vi "Init Platform Plugins.vi"(8 "error in (no error)":errorcluster, 11 "picoG in":refnum<class "picoG.lvclass">) -> (0 "error out":errorcluster, 3 "picoG out":refnum<class "picoG.lvclass">)   [LabVIEW 2020, in "PicoG-App.lvlib" / "picoG.lvclass"]
uses:
  picoG.lvclass
  picoG.lvclass/picoG.ctl
  Builds/picoG/ppl/PicoG-Core.lvlibp/PicoG-Processor/PicoG-Core/PlatformPluginManager/PlatformPluginManager.lvclass
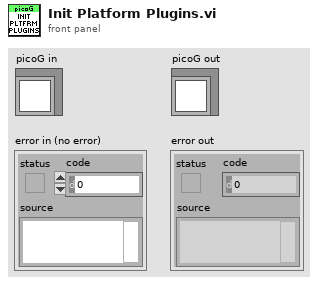
[diagram p1: front panel]
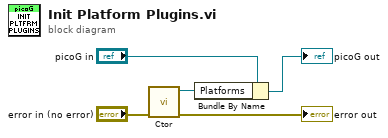
[diagram p0: block diagram]
diagram:
  n1 = call "Ctor.vi"("error in (no error)"="error in (no error)") -> ("error out"=→"error out":errorcluster, "TargetPluginManager out"=w4:refnum<class "PlatformPluginManager.lvclass">)  [unwired: 9 in]
  n2 = Bundle By Name(cluster="picoG in", "Platforms"=w4) -> (→"picoG out":refnum<class "picoG.lvclass">)
